vi "CheckCommandStartStop.vi"   [LabVIEW 2012]
types:
  T1 = cluster{"Name":string, "Parameters":string[], "Start Conditional":cluster{"String":string, "avgs":cluster{"Expression":string, "Durration":dbl, "Replacement":string, "Values":dbl[]}[]}, "End Conditional":cluster{"String":string, "avgs":cluster{"Expression":string, "Durration":dbl, "Replacement":string, "Values":dbl[]}[]}, "Running":bool}
  T2 = cluster{"String":string, "avgs":cluster{"Expression":string, "Durration":dbl, "Replacement":string, "Values":dbl[]}[]}
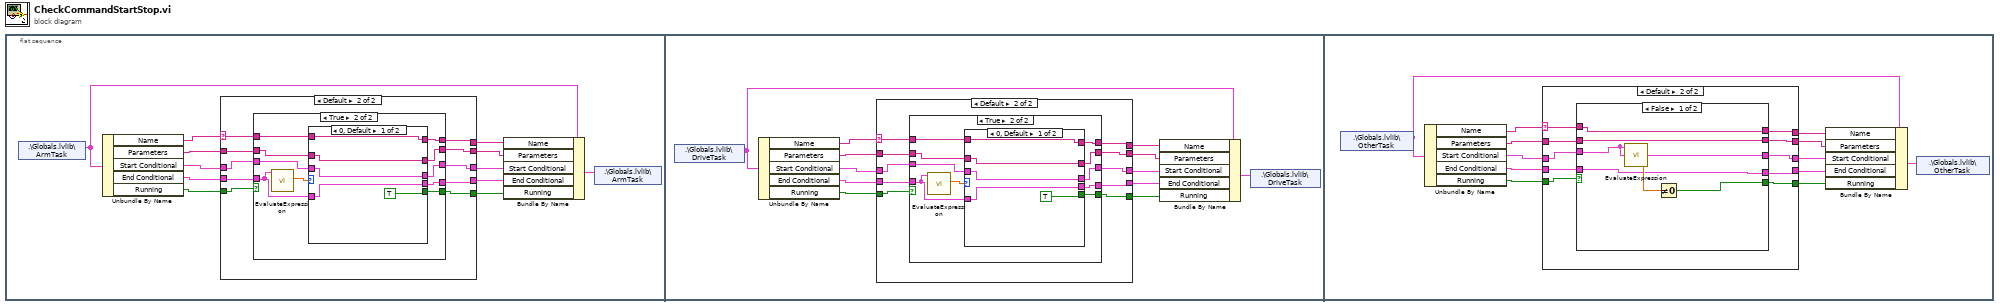
[diagram p0: block diagram]
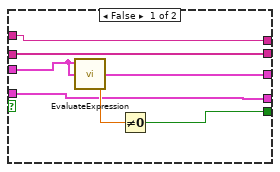
[diagram p3: hidden frame]
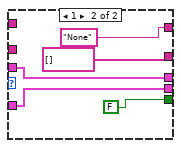
[diagram p4: hidden frame]
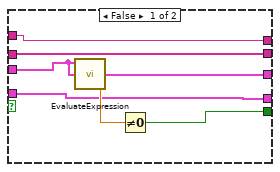
[diagram p6: hidden frame]
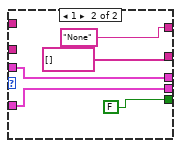
[diagram p7: hidden frame]
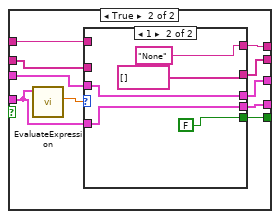
[diagram p9: hidden frame]
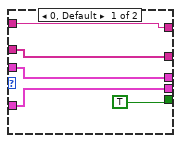
[diagram p10: hidden frame]
diagram:
  n1 = flat-sequence {
    frame #0 {
      n2 = shared-variable ".\\Globals.lvlib\\ArmTask"() -> (w9:T1)  [unwired: 1 in, 1 out]
      n3 = Unbundle By Name(w9) -> ("Name"=w7:string, "Parameters"=w11:string[], "Start Conditional"=w10:T2, "End Conditional"=w12:T2, "Running"=w6:bool)
      n4 = case shown="Default" w7 {
        selector: w7 -> [w16 w19]
        tunnel: w12 -> [w13 w24]
        tunnel: w11 -> [w15 w20]
        tunnel: w10 -> [w14 w25]
        tunnel: [w17 w26] -> w1
        tunnel: w6 -> [w17 w27]
        tunnel: [w16 w18] -> w5
        tunnel: [w15 w21] -> w4
        tunnel: [w14 w22] -> w3
        tunnel: [w13 w23] -> w2
        frame "None" {
        }
        frame Default {
          n5 = case shown="True" w27 {
            tunnel: [w32 w42] -> w26
            tunnel: w25 -> [w30 w39]
            tunnel: w24 -> [w31 w37]
            tunnel: [w31 w36] -> w23
            tunnel: [w30 w38] -> w22
            tunnel: w20 -> [w29 w35]
            tunnel: [w29 w40] -> w21
            tunnel: w19 -> [w28 w34]
            tunnel: [w28 w41] -> w18
            frame False {
              n6 = call "EvaluateExpression.vi"("Parsed Expression"=w30) -> ("Result"=w33:dbl)  [unwired: 9 in, 1 out]
              n7 = Not Equal To 0?(x=w33) -> (x != 0?=w32:bool)
            }
            frame True {
              n8 = call "EvaluateExpression.vi"("Parsed Expression"=w37) -> ("Result"=w43:dbl)  [unwired: 9 in, 1 out]
              n9 = case shown="0, Default" w43 {
                tunnel: [TRUE FALSE] -> w42
                tunnel: [w44 "None"] -> w41
                tunnel: [w45 string[] [] ("Parameters")] -> w40
                tunnel: w39 -> [w46 w50]
                tunnel: [w46 w50] -> w38
                tunnel: w37 -> [w47 w49]
                tunnel: [w47 w49] -> w36
                tunnel: w35 -> [w45 _]
                tunnel: w34 -> [w44 _]
                frame 0, Default {
                }
                frame 1 {
                }
              }
            }
          }
        }
      }
      n10 = Bundle By Name(cluster=w9, "Name"=w5, "Parameters"=w4, "Start Conditional"=w3, "End Conditional"=w2, "Running"=w1) -> (w8:T1)
      n11 = shared-variable ".\\Globals.lvlib\\ArmTask"(w8) -> ()  [unwired: 1 in, 1 out]
    }
    frame #1 {
      n12 = shared-variable ".\\Globals.lvlib\\DriveTask"() -> (w58:T1)  [unwired: 1 in, 1 out]
      n13 = Unbundle By Name(w58) -> ("Name"=w60:string, "Parameters"=w56:string[], "Start Conditional"=w57:T2, "End Conditional"=w55:T2, "Running"=w61:bool)
      n14 = case shown="Default" w60 {
        selector: w60 -> [w69 w72]
        tunnel: w55 -> [w66 w77]
        tunnel: w56 -> [w68 w73]
        tunnel: w57 -> [w67 w78]
        tunnel: [w70 w79] -> w54
        tunnel: w61 -> [w70 w80]
        tunnel: [w69 w71] -> w62
        tunnel: [w68 w74] -> w63
        tunnel: [w67 w75] -> w64
        tunnel: [w66 w76] -> w65
        frame "None" {
        }
        frame Default {
          n15 = case shown="True" w80 {
            tunnel: [w85 w95] -> w79
            tunnel: w78 -> [w83 w92]
            tunnel: w77 -> [w84 w90]
            tunnel: [w84 w89] -> w76
            tunnel: [w83 w91] -> w75
            tunnel: w73 -> [w82 w88]
            tunnel: [w82 w93] -> w74
            tunnel: w72 -> [w81 w87]
            tunnel: [w81 w94] -> w71
            frame False {
              n16 = call "EvaluateExpression.vi"("Parsed Expression"=w83) -> ("Result"=w86:dbl)  [unwired: 9 in, 1 out]
              n17 = Not Equal To 0?(x=w86) -> (x != 0?=w85:bool)
            }
            frame True {
              n18 = call "EvaluateExpression.vi"("Parsed Expression"=w90) -> ("Result"=w96:dbl)  [unwired: 9 in, 1 out]
              n19 = case shown="0, Default" w96 {
                tunnel: [TRUE FALSE] -> w95
                tunnel: [w97 "None"] -> w94
                tunnel: [w98 string[] [] ("Parameters")] -> w93
                tunnel: w92 -> [w99 w103]
                tunnel: [w99 w103] -> w91
                tunnel: w90 -> [w100 w102]
                tunnel: [w100 w102] -> w89
                tunnel: w88 -> [w98 _]
                tunnel: w87 -> [w97 _]
                frame 0, Default {
                }
                frame 1 {
                }
              }
            }
          }
        }
      }
      n20 = Bundle By Name(cluster=w58, "Name"=w62, "Parameters"=w63, "Start Conditional"=w64, "End Conditional"=w65, "Running"=w54) -> (w59:T1)
      n21 = shared-variable ".\\Globals.lvlib\\DriveTask"(w59) -> ()  [unwired: 1 in, 1 out]
    }
    frame #2 {
      n22 = shared-variable ".\\Globals.lvlib\\OtherTask"() -> (w115:T1)  [unwired: 1 in, 1 out]
      n23 = Unbundle By Name(w115) -> ("Name"=w113:string, "Parameters"=w117:string[], "Start Conditional"=w116:T2, "End Conditional"=w118:T2, "Running"=w112:bool)
      n24 = case shown="Default" w113 {
        selector: w113 -> [w122 w125]
        tunnel: w118 -> [w119 w130]
        tunnel: w117 -> [w121 w126]
        tunnel: w116 -> [w120 w131]
        tunnel: [w123 w132] -> w107
        tunnel: w112 -> [w123 w133]
        tunnel: [w122 w124] -> w111
        tunnel: [w121 w127] -> w110
        tunnel: [w120 w128] -> w109
        tunnel: [w119 w129] -> w108
        frame "None" {
        }
        frame Default {
          n25 = case shown="False" w133 {
            tunnel: [w138 w148] -> w132
            tunnel: w131 -> [w136 w145]
            tunnel: w130 -> [w137 w143]
            tunnel: [w137 w142] -> w129
            tunnel: [w136 w144] -> w128
            tunnel: w126 -> [w135 w141]
            tunnel: [w135 w146] -> w127
            tunnel: w125 -> [w134 w140]
            tunnel: [w134 w147] -> w124
            frame False {
              n26 = call "EvaluateExpression.vi"("Parsed Expression"=w136) -> ("Result"=w139:dbl)  [unwired: 9 in, 1 out]
              n27 = Not Equal To 0?(x=w139) -> (x != 0?=w138:bool)
            }
            frame True {
              n28 = call "EvaluateExpression.vi"("Parsed Expression"=w143) -> ("Result"=w149:dbl)  [unwired: 9 in, 1 out]
              n29 = case shown="1" w149 {
                tunnel: [TRUE FALSE] -> w148
                tunnel: [w150 "None"] -> w147
                tunnel: [w151 string[] [] ("Parameters")] -> w146
                tunnel: w145 -> [w152 w156]
                tunnel: [w152 w156] -> w144
                tunnel: w143 -> [w153 w155]
                tunnel: [w153 w155] -> w142
                tunnel: w141 -> [w151 _]
                tunnel: w140 -> [w150 _]
                frame 0, Default {
                }
                frame 1 {
                }
              }
            }
          }
        }
      }
      n30 = Bundle By Name(cluster=w115, "Name"=w111, "Parameters"=w110, "Start Conditional"=w109, "End Conditional"=w108, "Running"=w107) -> (w114:T1)
      n31 = shared-variable ".\\Globals.lvlib\\OtherTask"(w114) -> ()  [unwired: 1 in, 1 out]
    }
  }
